vi "cleanupLaserHW.vi"(8 "error in (no error)":errorcluster) -> (0 "error out":errorcluster)   [LabVIEW 2012]
uses:
  bin/OVA32.dll
panel:
  out "DLL Return Code":i32
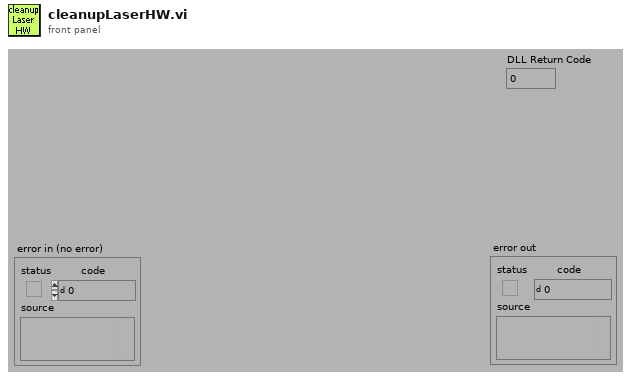
[diagram p1: front panel]
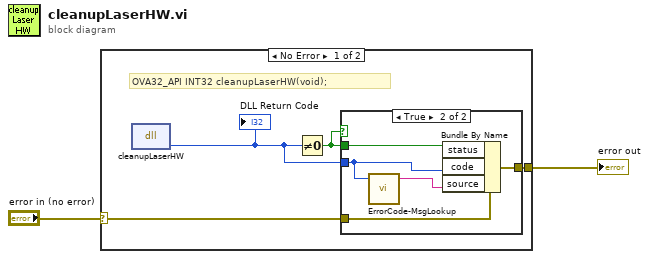
[diagram p0: block diagram]
diagram:
  n1 = case shown="No Error" "error in (no error)" {
    selector: "error in (no error)" -> [w3 w13]
    tunnel: [w6 w13] -> w2
    frame No Error {
      # "OVA32_API INT32 cleanupLaserHW(void);"
      n2 = dll-call lib="C:/_src/OVA5000_DSP_falcon/Software/LabVIEW/OVA/SDK/OVA_5000_SDK_v5.14.3/bin/OVA32.dll" fn="cleanupLaserHW"() -> (w5:u8)  [unwired: 3 in, 2 out]
      "DLL Return Code" <- w5
      n3 = Not Equal To 0?(x=w5) -> (x != 0?=w4:bool)
      n4 = case shown="True" w4 {
        tunnel: w3 -> [w7 w12]
        tunnel: w4 -> [_ w11]
        tunnel: [w7 w10] -> w6
        tunnel: w5 -> [_ w9]
        frame False {
        }
        frame True {
          n5 = call "ErrorCode-MsgLookup.vi"("DLL Return Code"=w9) -> ("Error String"=w8:string)  [unwired: 2 in, 2 out]
          n6 = Bundle By Name(cluster=w12, "status"=w11, "code"=w9, "source"=w8) -> (w10:errorcluster)
        }
      }
    }
    frame Error {
    }
  }
  "error out" <- w2
